vi "libssh2_agent_init.vi"(8 "error in (no error)":errorcluster, 11 "session":T1) -> (0 "error out":errorcluster, 3 "agent":T2)   [LabVIEW 2013, in "libssh2.lvlib"]
doc: "Initialize an SSH agent handle. The caller is responsible for releasing the handle by calling <B>libssh2_agent_free</B>."
uses:
  libssh2.lvlib
  Agent Refnum.ctl
  Session Refnum.ctl
  Not A Session.vi
  <vilib>/Utility/error.llb/Error Cluster From Error Code.vi
  Global Settings.vi
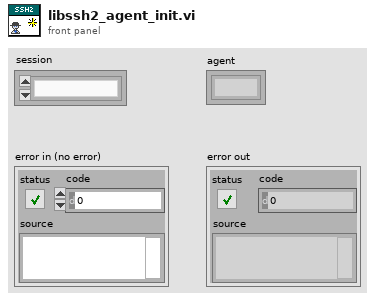
[diagram p1: front panel]
types:
  T1 = typedef "libssh2.lvlib/Session Refnum.ctl" = refnum<k1>
  T2 = typedef "libssh2.lvlib/Agent Refnum.ctl" = refnum<k1>
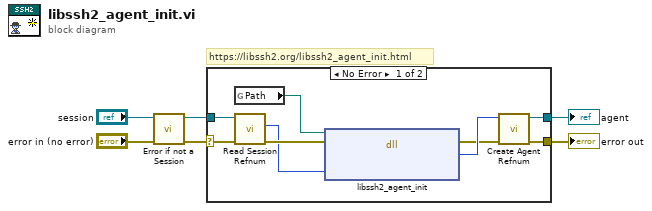
[diagram p0: block diagram]
diagram:
  # "https://libssh2.org/libssh2_agent_init.html"
  n1 = call "Error if not a Session.vi"("error in (no error)"="error in (no error)", "session"="session") -> ("error out"=w3:errorcluster, "session out"=w2:T1)  [unwired: 8 in]
  n2 = case shown="No Error" w3 {
    selector: w3 -> [w13 w16]
    tunnel: [w15 _] -> w4
    tunnel: [w14 w16] -> w6
    tunnel: w2 -> [w12 _]
    frame No Error {
      n3 = global read "Global Settings.vi" "Path"() -> (w9:path)
      n4 = call "Read Session Refnum.vi"("error in (no error)"=w13, "session"=w12) -> ("error out"=w8:errorcluster, "LIBSSH2_SESSION*"=w7:u64)  [unwired: 5 in, 3 out]
      n5 = dll-call lib="?" fn="libssh2_agent_init"(path in=w9, error in=w8, "session"=w7) -> (error out=w10:errorcluster, "return value"=w11:u64)  [unwired: 2 in, 1 out]
      n6 = call "Create Agent Refnum.vi"("error in (no error)"=w10, "LIBSSH2_AGENT*"=w11) -> ("error out"=w14:errorcluster, "agent"=w15:T2)  [unwired: 8 in]
    }
    frame Error {
    }
  }
  "error out" <- w6
  "agent" <- w4
